vi "webBrowser.vi"(11 "Automation Refnum in":refnum<k7>(container)) -> ()   [LabVIEW 2014]
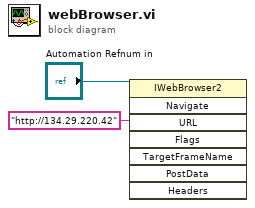
[diagram p0: block diagram]
diagram:
  n1 = invoke class="IWebBrowser2" method="Navigate"(reference="Automation Refnum in", "URL"="http://134.29.220.42") -> ()  [unwired: 6 in, 8 out]
